vi "Border_171213.vi"(9 "StartingAngle":i16=120, 10 "Border":enum16{"8", "6", "5", "4", "3", "2", "1", "0"}(ring), 11 "InputBackground":picture) -> (2 "Colors":u32[](array[numeric]), 3 "OutputPicture":picture)   [LabVIEW 2016]
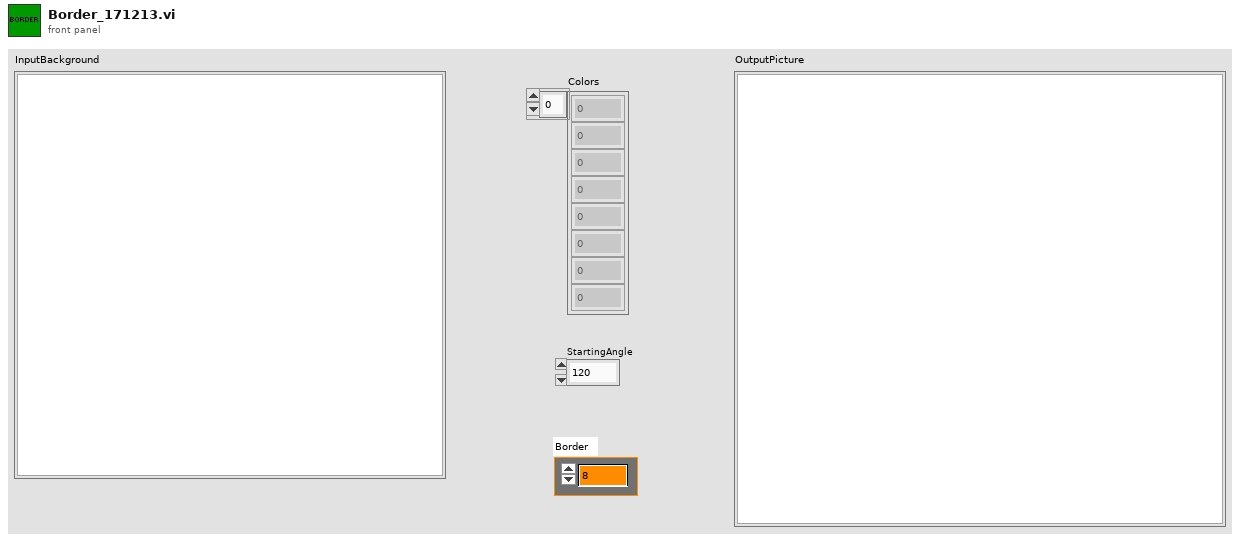
[diagram p1: front panel]
types:
  T1 = cluster{"left":i16, "top":i16, "right":i16, "bottom":i16}
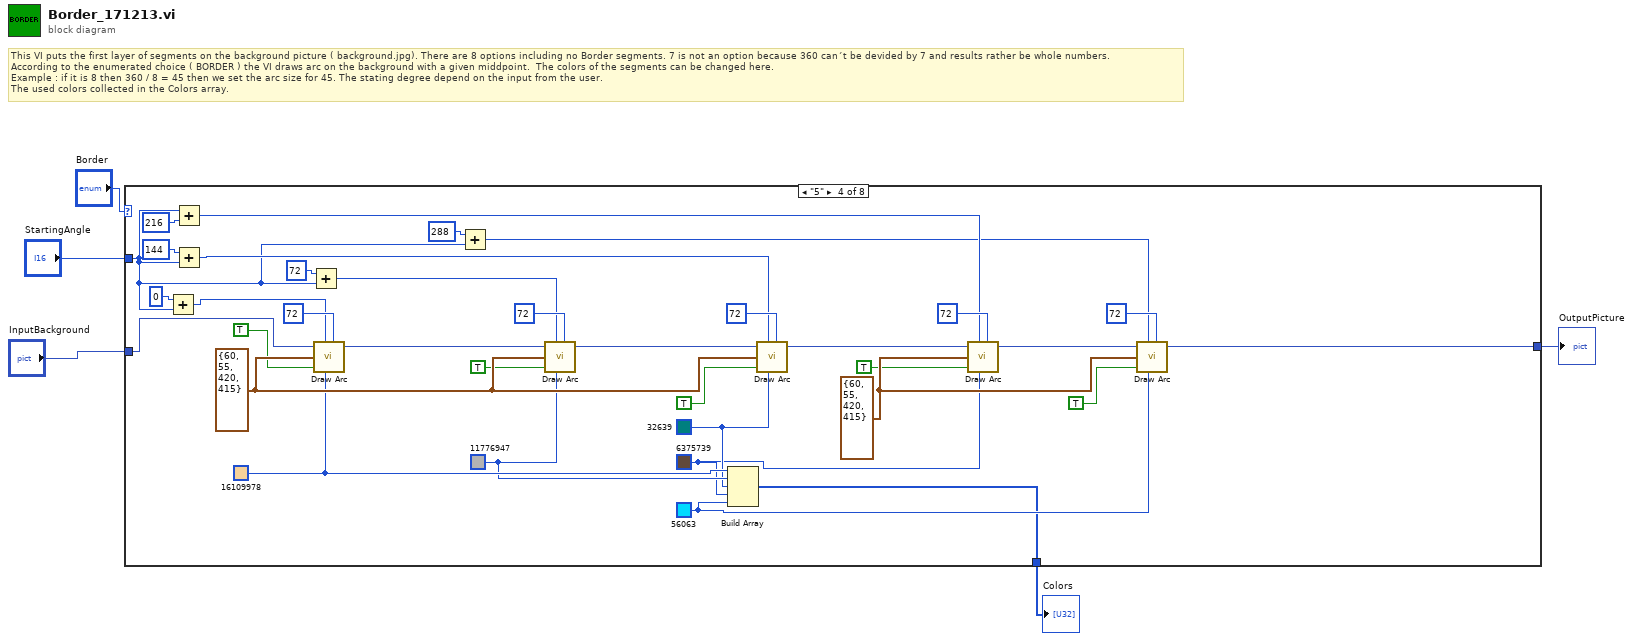
[diagram p0: block diagram]
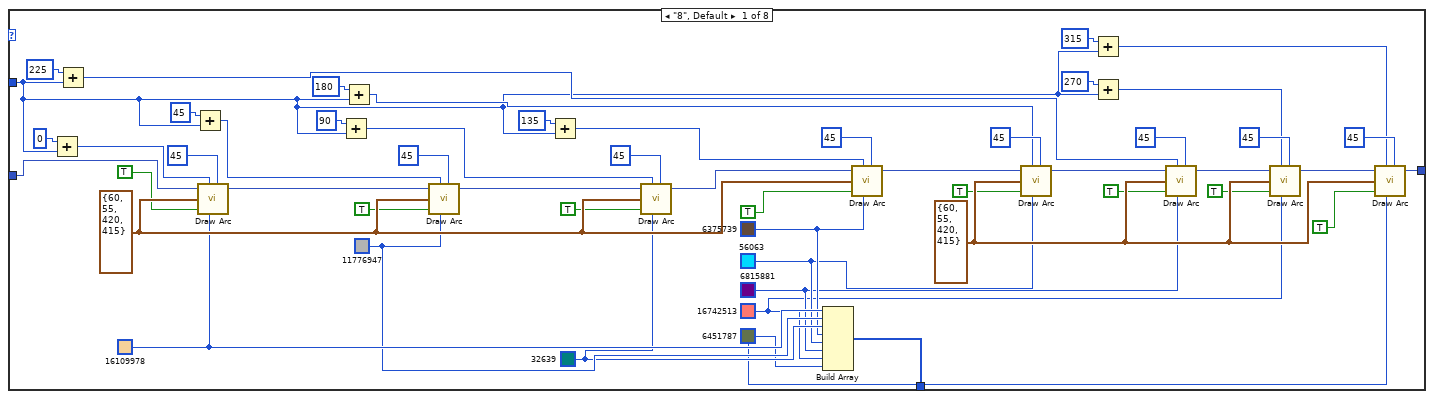
[diagram p2: hidden frame]
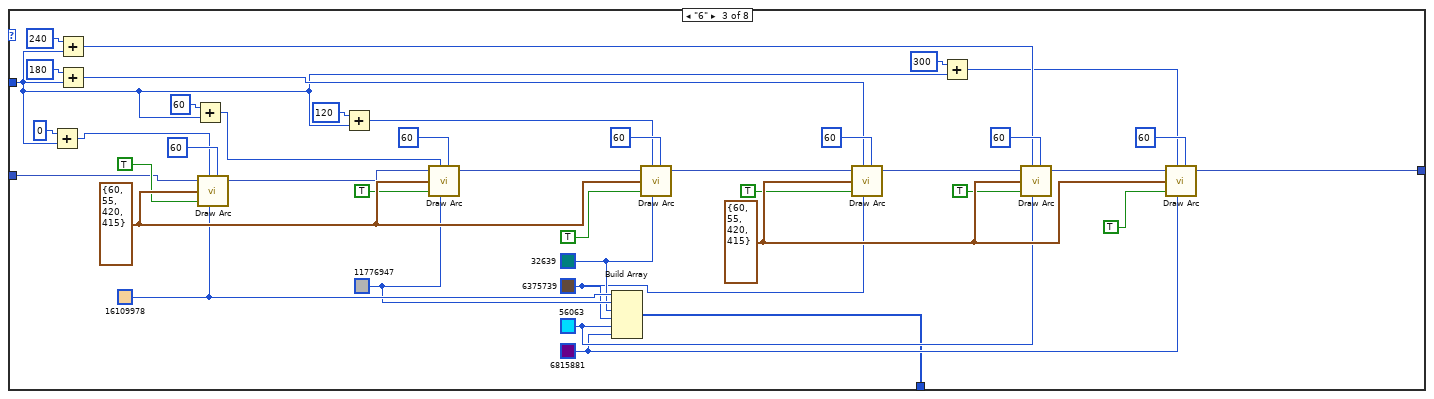
[diagram p4: hidden frame]
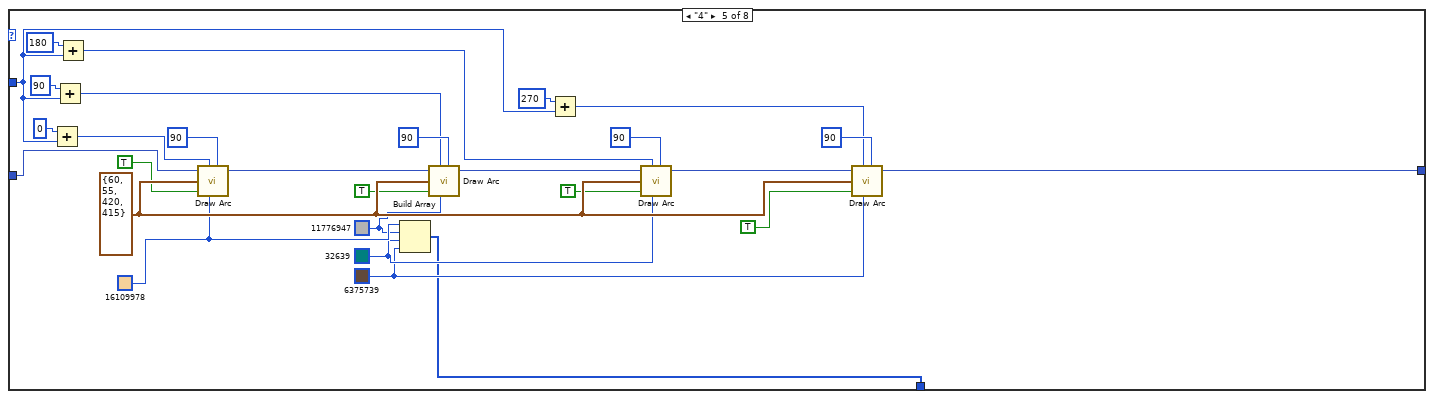
[diagram p5: hidden frame]
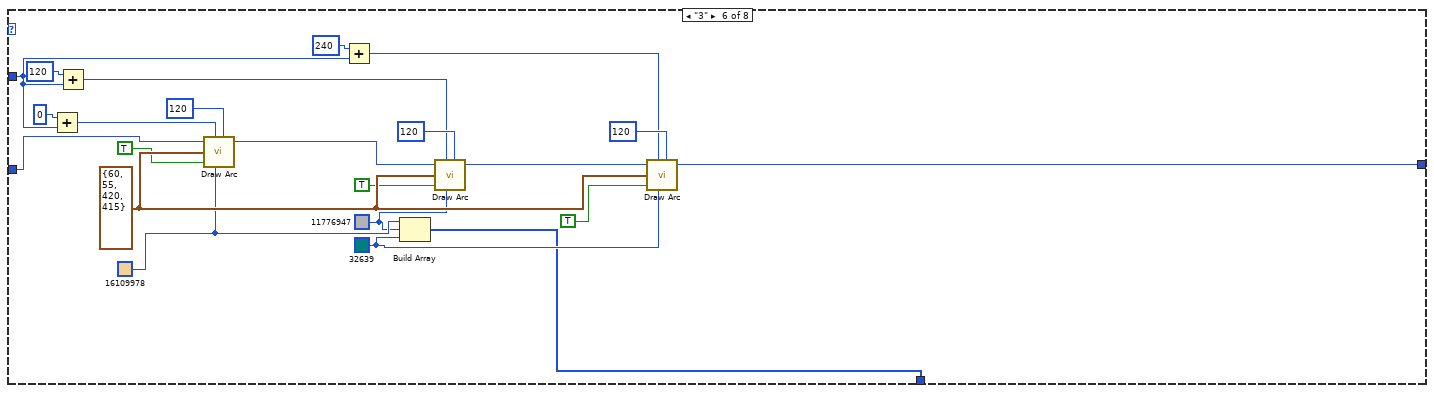
[diagram p6: hidden frame]
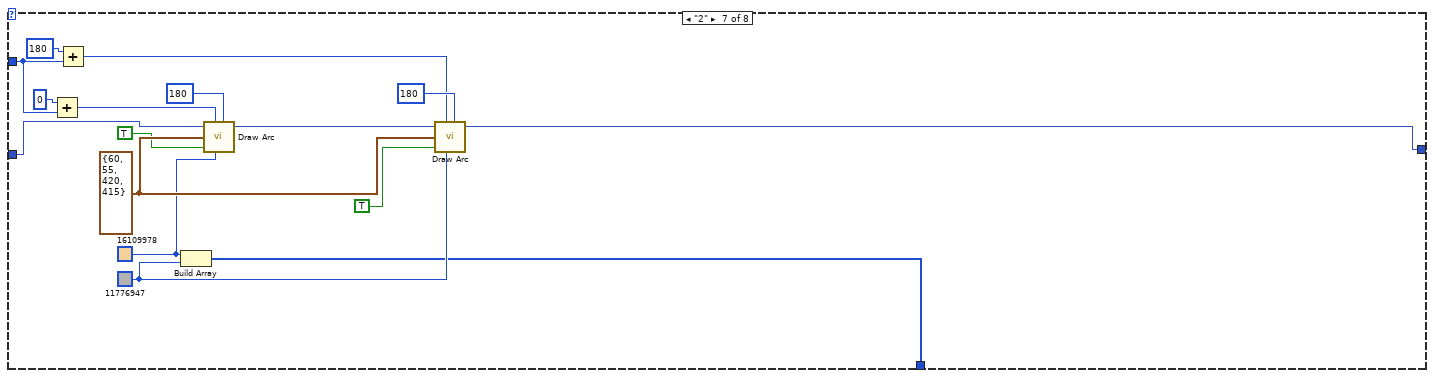
[diagram p7: hidden frame]
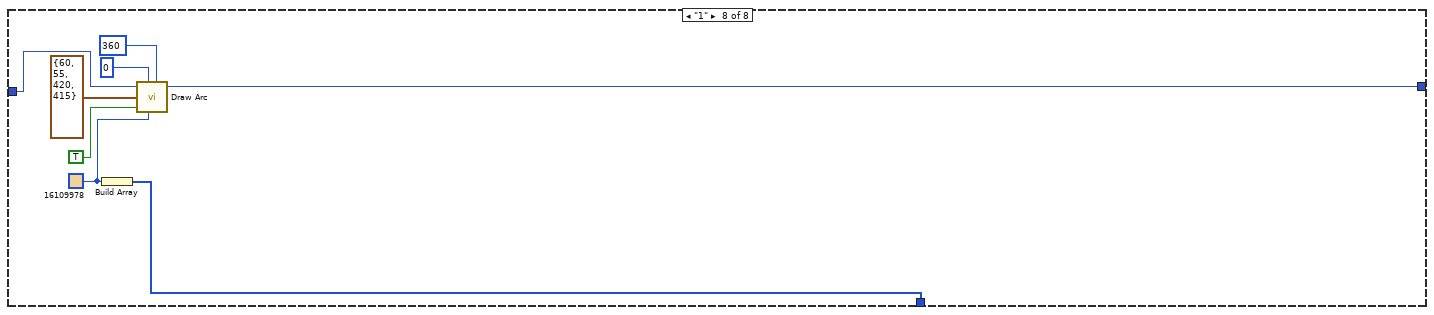
[diagram p8: hidden frame]
diagram:
  # "This VI puts the first layer of segments on the background picture ( background.jpg). There are 8 options including no Border segments. 7 is not an option because 360 can´t be devided by 7 and results rather be whole numbers. \nAccording to the enumerated choice ( BORDER ) the VI draws arc on the background with a given middpoint.  The colors of the segments can be changed here. \nExample : if it is 8 then 360 / 8 = 45 then we set the arc size for 45. The stating degree depend on the input from the user. \nThe used colors collected in the Colors array."
  n1 = case shown="\"5\"" "Border" {
    tunnel: "InputBackground" -> [w27 w59 w74 w114 w147 w173 w194 w205]
    tunnel: [w25 w59 w75 w113 w146 w172 w193 w204] -> w4
    tunnel: "StartingAngle" -> [w7 _ w61 w102 w137 w165 w187 _]
    tunnel: [w6 _ w60 w101 w136 w164 w186 w202] -> w1
    frame "8", Default {
      w16 = u32 6451787 ("color(black)")
      w17 = u32 16742513 ("color(black)")
      w18 = u32 6815881 ("color(black)")
      w19 = u32 56063 ("color(black)")
      w43 = T1 {"left"=60, "top"=55, "right"=420, "bottom"=415} ("rect")
      w20 = u32 6375739 ("color(black)")
      w21 = u32 32639 ("color(black)")
      w22 = u32 11776947 ("color(black)")
      w23 = u32 16109978 ("color(black)")
      w58 = T1 {"left"=60, "top"=55, "right"=420, "bottom"=415} ("rect")
      n2 = Add(x=i16 0 ("start angle[degrees]"), y=w7) -> (x+y=w15:i16)
      n3 = Add(x=i16 225 ("start angle[degrees]"), y=w7) -> (x+y=w10:i16)
      n4 = Add(x=i16 45 ("start angle[degrees]"), y=w7) -> (x+y=w14:i16)
      n5 = call <vilib>:"Draw Arc.vi"("picture"=w27, "start angle[degrees]"=w15, "rect"=w58, "fill?(F)"=TRUE, "color(black)"=w23, "arc size[degrees]"=i16 45) -> ("new picture"=w50:picture)  [unwired: 3 in]
      n6 = Add(x=i16 90 ("start angle[degrees]"), y=w7) -> (x+y=w13:i16)
      n7 = Add(x=i16 180 ("start angle[degrees]"), y=w7) -> (x+y=w11:i16)
      n8 = call <vilib>:"Draw Arc.vi"("picture"=w50, "start angle[degrees]"=w14, "rect"=w58, "fill?(F)"=TRUE, "color(black)"=w22, "arc size[degrees]"=i16 45) -> ("new picture"=w54:picture)  [unwired: 3 in]
      n9 = Add(x=i16 135 ("start angle[degrees]"), y=w7) -> (x+y=w12:i16)
      n10 = call <vilib>:"Draw Arc.vi"("picture"=w54, "start angle[degrees]"=w13, "rect"=w58, "fill?(F)"=TRUE, "color(black)"=w21, "arc size[degrees]"=i16 45) -> ("new picture"=w57:picture)  [unwired: 3 in]
      n11 = Build Array(w23, w22, w21, w20, w19, w18, w17, w16) -> (w6:u32[])
      n12 = call <vilib>:"Draw Arc.vi"("picture"=w57, "start angle[degrees]"=w12, "rect"=w58, "fill?(F)"=TRUE, "color(black)"=w20, "arc size[degrees]"=i16 45) -> ("new picture"=w26:picture)  [unwired: 3 in]
      n13 = call <vilib>:"Draw Arc.vi"("picture"=w26, "start angle[degrees]"=w11, "rect"=w43, "fill?(F)"=TRUE, "color(black)"=w19, "arc size[degrees]"=i16 45) -> ("new picture"=w34:picture)  [unwired: 3 in]
      n14 = Add(x=i16 315 ("start angle[degrees]"), y=w7) -> (x+y=w8:i16)
      n15 = Add(x=i16 270 ("start angle[degrees]"), y=w7) -> (x+y=w9:i16)
      n16 = call <vilib>:"Draw Arc.vi"("picture"=w34, "start angle[degrees]"=w10, "rect"=w43, "fill?(F)"=TRUE, "color(black)"=w18, "arc size[degrees]"=i16 45) -> ("new picture"=w38:picture)  [unwired: 3 in]
      n17 = call <vilib>:"Draw Arc.vi"("picture"=w38, "start angle[degrees]"=w9, "rect"=w43, "fill?(F)"=TRUE, "color(black)"=w17, "arc size[degrees]"=i16 45) -> ("new picture"=w42:picture)  [unwired: 3 in]
      n18 = call <vilib>:"Draw Arc.vi"("picture"=w42, "start angle[degrees]"=w8, "rect"=w43, "fill?(F)"=TRUE, "color(black)"=w16, "arc size[degrees]"=i16 45) -> ("new picture"=w25:picture)  [unwired: 3 in]
    }
    frame "0" {
    }
    frame "6" {
      w68 = u32 6815881 ("color(black)")
      w69 = u32 56063 ("color(black)")
      w70 = u32 6375739 ("color(black)")
      w88 = T1 {"left"=60, "top"=55, "right"=420, "bottom"=415} ("rect")
      w71 = u32 32639 ("color(black)")
      w72 = u32 11776947 ("color(black)")
      w73 = u32 16109978 ("color(black)")
      w100 = T1 {"left"=60, "top"=55, "right"=420, "bottom"=415} ("rect")
      n19 = Add(x=i16 0 ("start angle[degrees]"), y=w61) -> (x+y=w67:i16)
      n20 = Add(x=i16 240 ("start angle[degrees]"), y=w61) -> (x+y=w63:i16)
      n21 = Add(x=i16 180 ("start angle[degrees]"), y=w61) -> (x+y=w64:i16)
      n22 = Add(x=i16 60 ("start angle[degrees]"), y=w61) -> (x+y=w66:i16)
      n23 = call <vilib>:"Draw Arc.vi"("picture"=w74, "start angle[degrees]"=w67, "rect"=w100, "fill?(F)"=TRUE, "color(black)"=w73, "arc size[degrees]"=i16 60) -> ("new picture"=w95:picture)  [unwired: 3 in]
      n24 = Add(x=i16 120 ("start angle[degrees]"), y=w61) -> (x+y=w65:i16)
      n25 = call <vilib>:"Draw Arc.vi"("picture"=w95, "start angle[degrees]"=w66, "rect"=w100, "fill?(F)"=TRUE, "color(black)"=w72, "arc size[degrees]"=i16 60) -> ("new picture"=w99:picture)  [unwired: 3 in]
      n26 = Build Array(w73, w72, w71, w70, w69, w68) -> (w60:u32[])
      n27 = call <vilib>:"Draw Arc.vi"("picture"=w99, "start angle[degrees]"=w65, "rect"=w100, "fill?(F)"=TRUE, "color(black)"=w71, "arc size[degrees]"=i16 60) -> ("new picture"=w76:picture)  [unwired: 3 in]
      n28 = call <vilib>:"Draw Arc.vi"("picture"=w76, "start angle[degrees]"=w64, "rect"=w88, "fill?(F)"=TRUE, "color(black)"=w70, "arc size[degrees]"=i16 60) -> ("new picture"=w83:picture)  [unwired: 3 in]
      n29 = Add(x=i16 300 ("start angle[degrees]"), y=w61) -> (x+y=w62:i16)
      n30 = call <vilib>:"Draw Arc.vi"("picture"=w83, "start angle[degrees]"=w63, "rect"=w88, "fill?(F)"=TRUE, "color(black)"=w69, "arc size[degrees]"=i16 60) -> ("new picture"=w87:picture)  [unwired: 3 in]
      n31 = call <vilib>:"Draw Arc.vi"("picture"=w87, "start angle[degrees]"=w62, "rect"=w88, "fill?(F)"=TRUE, "color(black)"=w68, "arc size[degrees]"=i16 60) -> ("new picture"=w75:picture)  [unwired: 3 in]
    }
    frame "5" {
      w108 = u32 56063 ("color(black)")
      w109 = u32 6375739 ("color(black)")
      w110 = u32 32639 ("color(black)")
      w111 = u32 11776947 ("color(black)")
      w112 = u32 16109978 ("color(black)")
      w123 = T1 {"left"=60, "top"=55, "right"=420, "bottom"=415} ("rect")
      w135 = T1 {"left"=60, "top"=55, "right"=420, "bottom"=415} ("rect")
      n32 = Add(x=i16 0 ("start angle[degrees]"), y=w102) -> (x+y=w107:i16)
      n33 = Add(x=w102, y=i16 216 ("start angle[degrees]")) -> (x+y=w104:i16)
      n34 = Add(x=i16 144 ("start angle[degrees]"), y=w102) -> (x+y=w105:i16)
      n35 = Add(x=i16 72 ("start angle[degrees]"), y=w102) -> (x+y=w106:i16)
      n36 = call <vilib>:"Draw Arc.vi"("picture"=w114, "start angle[degrees]"=w107, "rect"=w135, "fill?(F)"=TRUE, "color(black)"=w112, "arc size[degrees]"=i16 72) -> ("new picture"=w130:picture)  [unwired: 3 in]
      n37 = Add(x=i16 288 ("start angle[degrees]"), y=w102) -> (x+y=w103:i16)
      n38 = call <vilib>:"Draw Arc.vi"("picture"=w130, "start angle[degrees]"=w106, "rect"=w135, "fill?(F)"=TRUE, "color(black)"=w111, "arc size[degrees]"=i16 72) -> ("new picture"=w134:picture)  [unwired: 3 in]
      n39 = Build Array(w112, w111, w110, w109, w108) -> (w101:u32[])
      n40 = call <vilib>:"Draw Arc.vi"("picture"=w134, "start angle[degrees]"=w105, "rect"=w135, "fill?(F)"=TRUE, "color(black)"=w110, "arc size[degrees]"=i16 72) -> ("new picture"=w115:picture)  [unwired: 3 in]
      n41 = call <vilib>:"Draw Arc.vi"("picture"=w115, "start angle[degrees]"=w104, "rect"=w123, "fill?(F)"=TRUE, "color(black)"=w109, "arc size[degrees]"=i16 72) -> ("new picture"=w122:picture)  [unwired: 3 in]
      n42 = call <vilib>:"Draw Arc.vi"("picture"=w122, "start angle[degrees]"=w103, "rect"=w123, "fill?(F)"=TRUE, "color(black)"=w108, "arc size[degrees]"=i16 72) -> ("new picture"=w113:picture)  [unwired: 3 in]
    }
    frame "4" {
      w142 = u32 6375739 ("color(black)")
      w143 = u32 32639 ("color(black)")
      w144 = u32 11776947 ("color(black)")
      w145 = u32 16109978 ("color(black)")
      w163 = T1 {"left"=60, "top"=55, "right"=420, "bottom"=415} ("rect")
      n43 = Add(x=i16 0 ("start angle[degrees]"), y=w137) -> (x+y=w141:i16)
      n44 = Add(x=i16 90 ("start angle[degrees]"), y=w137) -> (x+y=w140:i16)
      n45 = Add(x=i16 180 ("start angle[degrees]"), y=w137) -> (x+y=w139:i16)
      n46 = call <vilib>:"Draw Arc.vi"("picture"=w147, "start angle[degrees]"=w141, "rect"=w163, "fill?(F)"=TRUE, "color(black)"=w145, "arc size[degrees]"=i16 90) -> ("new picture"=w158:picture)  [unwired: 3 in]
      n47 = Build Array(w145, w144, w143, w142) -> (w136:u32[])
      n48 = call <vilib>:"Draw Arc.vi"("picture"=w158, "start angle[degrees]"=w140, "rect"=w163, "fill?(F)"=TRUE, "color(black)"=w144, "arc size[degrees]"=i16 90) -> ("new picture"=w162:picture)  [unwired: 3 in]
      n49 = Add(x=i16 270 ("start angle[degrees]"), y=w137) -> (x+y=w138:i16)
      n50 = call <vilib>:"Draw Arc.vi"("picture"=w162, "start angle[degrees]"=w139, "rect"=w163, "fill?(F)"=TRUE, "color(black)"=w143, "arc size[degrees]"=i16 90) -> ("new picture"=w148:picture)  [unwired: 3 in]
      n51 = call <vilib>:"Draw Arc.vi"("picture"=w148, "start angle[degrees]"=w138, "rect"=w163, "fill?(F)"=TRUE, "color(black)"=w142, "arc size[degrees]"=i16 90) -> ("new picture"=w146:picture)  [unwired: 3 in]
    }
    frame "3" {
      w169 = u32 32639 ("color(black)")
      w170 = u32 11776947 ("color(black)")
      w171 = u32 16109978 ("color(black)")
      w185 = T1 {"left"=60, "top"=55, "right"=420, "bottom"=415} ("rect")
      n52 = Add(x=i16 0 ("start angle[degrees]"), y=w165) -> (x+y=w168:i16)
      n53 = Add(x=i16 120 ("start angle[degrees]"), y=w165) -> (x+y=w167:i16)
      n54 = call <vilib>:"Draw Arc.vi"("picture"=w173, "start angle[degrees]"=w168, "rect"=w185, "fill?(F)"=TRUE, "color(black)"=w171, "arc size[degrees]"=i16 120) -> ("new picture"=w180:picture)  [unwired: 3 in]
      n55 = Add(x=i16 240 ("start angle[degrees]"), y=w165) -> (x+y=w166:i16)
      n56 = Build Array(w171, w170, w169) -> (w164:u32[])
      n57 = call <vilib>:"Draw Arc.vi"("picture"=w180, "start angle[degrees]"=w167, "rect"=w185, "fill?(F)"=TRUE, "color(black)"=w170, "arc size[degrees]"=i16 120) -> ("new picture"=w184:picture)  [unwired: 3 in]
      n58 = call <vilib>:"Draw Arc.vi"("picture"=w184, "start angle[degrees]"=w166, "rect"=w185, "fill?(F)"=TRUE, "color(black)"=w169, "arc size[degrees]"=i16 120) -> ("new picture"=w172:picture)  [unwired: 3 in]
    }
    frame "2" {
      w191 = u32 11776947 ("color(black)")
      w192 = u32 16109978 ("color(black)")
      w201 = T1 {"left"=60, "top"=55, "right"=420, "bottom"=415} ("rect")
      n59 = Add(x=i16 0 ("start angle[degrees]"), y=w187) -> (x+y=w189:i16)
      n60 = Add(x=i16 180 ("start angle[degrees]"), y=w187) -> (x+y=w188:i16)
      n61 = Build Array(w192, w191) -> (w186:u32[])
      n62 = call <vilib>:"Draw Arc.vi"("picture"=w194, "start angle[degrees]"=w189, "rect"=w201, "fill?(F)"=TRUE, "color(black)"=w192, "arc size[degrees]"=i16 180) -> ("new picture"=w200:picture)  [unwired: 3 in]
      n63 = call <vilib>:"Draw Arc.vi"("picture"=w200, "start angle[degrees]"=w188, "rect"=w201, "fill?(F)"=TRUE, "color(black)"=w191, "arc size[degrees]"=i16 180) -> ("new picture"=w193:picture)  [unwired: 3 in]
    }
    frame "1" {
      w203 = u32 16109978 ("color(black)")
      n64 = Build Array(w203) -> (w202:u32[])
      n65 = call <vilib>:"Draw Arc.vi"("picture"=w205, "start angle[degrees]"=i16 0, "rect"=T1 {"left"=60, "top"=55, "right"=420, "bottom"=415}, "fill?(F)"=TRUE, "color(black)"=w203, "arc size[degrees]"=i16 360) -> ("new picture"=w204:picture)  [unwired: 3 in]
    }
  }
  "OutputPicture" <- w4
  "Colors" <- w1
